vi "music reconstruct(SubVI).vi"(10 "path":path, 11 "output bit stream in":i8[](array[numeric]) caption="output bit stream") -> ()   [LabVIEW 2026]
uses:
  <vilib>/sound2/lvsound2.llb/Sound File Write (DBL Single).vi
  <vilib>/sound2/lvsound2.llb/Sound File Write Open.vi
  <vilib>/sound2/lvsound2.llb/Sound File Info (path).vi
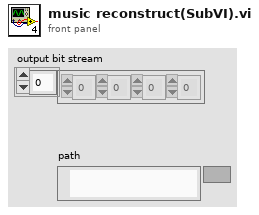
[diagram p1: front panel]
types:
  T1 = typedef "Sound Data Format.ctl" = cluster{"sample rate (S/s)":dbl, "number of channels":i32, "bits per sample":i32}
  T2 = typedef "Sound File Refnum.ctl" = refnum<file>
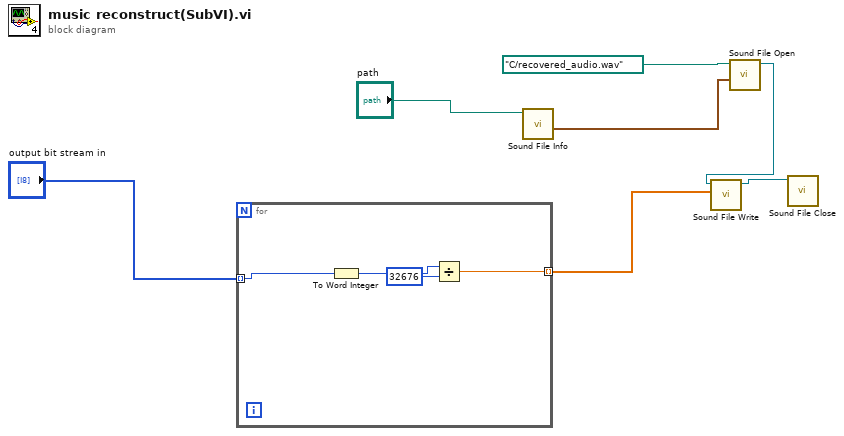
[diagram p0: block diagram]
diagram:
  n1 = for {
    tunnel: "output bit stream in" -> [w11] mode=indexing
    tunnel: [w8] -> w4 mode=indexing
    n2 = To Word Integer(number=w11) -> (16bit integer=w10:i16)
    n3 = Divide(x=w10, y=i16 32676) -> (x/y=w8:dbl)
  }
  n4 = call-poly <vilib>:"Sound File Info.vi"("path"="path") -> ("sound format"=w6:T1)  [unwired: 7 in, 3 out]
  n5 = call-poly <vilib>:"Sound File Open.vi"("sound format"=w6, "path"=path "C:/recovered_audio.wav") -> ("sound file refnum"=w2:T2)  [unwired: 8 in, 1 out]
  n6 = call-poly <vilib>:"Sound File Write.vi"("data"=w4, "sound file refnum"=w2) -> ("sound file refnum out"=w1:T2)  [unwired: 8 in, 1 out]
  n7 = call <vilib>:"Sound File Close.vi"("sound file refnum"=w1) -> ()  [unwired: 10 in, 1 out]
